vi "PH_HamamatsuCamera.ProcPeriodic.vi"(0 "i ref in":refnum<vi>, 3 "ms timeout (100)":i32=100, 5 "error in (no error)":errorcluster) -> (14 "i ref out":refnum<vi>, 17 "timed out":bool, 19 "error out":errorcluster)   [LabVIEW 2014, in "PH_HamamatsuCamera.lvlib"]
doc: "This method serves to periodically do things like reading values from the HW. Methods that should be executed periodically should be called from THIS methode. Add code here."
uses:
  PH_HamamatsuCamera.lvlib
  PH_StatusHandler/PH_StatusHandler.Status.ctl
  PH_Cam_BaseClass/PH_Cam_BaseClass.lvlib
  CSCore/BaseProcess/BaseProcess.lvlib
  PH_StatusHandler/PH_StatusHandler.lvlib
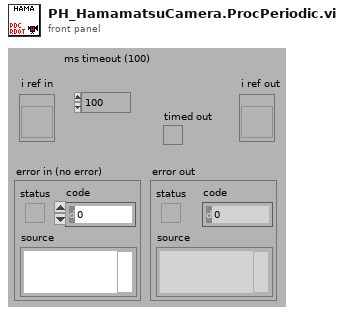
[diagram p1: front panel]
types:
  T1 = typedef "PH_Cam_BaseClass.lvlib/PH_Cam_BaseClass.i attribute.ctl" = cluster{"Gui Refs":T2, "Cam":cluster{"Source Notifier":refnum<notifier>, "Error":errorcluster, "Camera ID":string}, "Images":cluster{"Cam":T3, "Operation":T3, "PSDB":T3}, "Window Image":cluster{"Indicate Image":bool, "Window No.":i32, "Scale Facor":dbl, "Center Cross":bool, "Subtract Backgr":bool, "CoG":bool, "Color Palette":cluster{"Red":u8, "Green":u8, "Blue":u8}[], "Image On":bool}, "Default Prdc Int":i32, "Performance":cluster{"on":bool, "Timestamp Last Frame":i32}, "Histogram":cluster{"on":bool, "Mapping":bool}, "Save Image":cluster{"Save":bool, "File refnum":refnum<file>}, "Setting Service ID":i32, "Screen":cluster{"x-resolution":i16, "y-resolution":i16}, "On":bool, "Constructor finished":bool, "configured":bool}
  T2 = typedef "PH_Cam_BaseClass.lvlib/PH_Cam_BaseClass.GUI Refs.ctl" = cluster{"Frame Rate":refnum<vi>, "Get Frame Rate":refnum<vi>, "Show Image":refnum<vi>, "Get Histogram":refnum<vi>, "Mapping":refnum<vi>, "Histogram":refnum<vi>, "Center Cross":refnum<vi>, "Center of Gravity":refnum<vi>, "Scale Factor [%]":refnum<vi>, "Save Image":refnum<vi>, "Palette":refnum<vi>, "Subtract Background":refnum<vi>, "Cam Error":refnum<vi>, "On":refnum<vi>, "Cam List":refnum<vi>}
  T3 = typedef "IMAQ Image.ctl" = refnum<image>
  T4 = typedef "PH_StatusHandler.lvlib/PH_StatusHandler.Status.ctl" = i16
  T5 = typedef "PH_Cam_BaseClass.lvlib/PH_Cam_BaseClass.Settings.ctl" = cluster{"Cam ID":string, "Gain":dbl, "Brightness":dbl, "Shutter":dbl, "Mode":i32}
  T6 = typedef "PH_HamamatsuCamera.lvlib/PH_HamamatsuCamera.i attribute.ctl" = cluster{"Gui Refs":cluster{"Camera Details":refnum<vi>, "ROI":refnum<vi>, "Set ROI to Maximum":refnum<vi>, "Trigger Parameters":refnum<vi>, "Brightness":refnum<vi>, "Shutter":refnum<vi>, "Gain":refnum<vi>, "Trigger Timeout":refnum<vi>, "Trigger Polarity":refnum<vi>, "Trigger Mode":refnum<vi>, "Parameters":refnum<vi>, "Set Cam Parameter":refnum<vi>, "Parameter to set":refnum<vi>, "Value to set":refnum<vi>}, "Cam":cluster{"Handle":i32, "Details":cluster{"Model":string, "Camera ID":string, "Firmware":string}, "Buffer Info":cluster{"height":u32, "width":u32, "datatype":u32}}, "H Offset":cluster{"Value":i32, "Minimum":i32, "Maximum":i32, "Increment":i32}, "V Offset":cluster{"Value":i32, "Minimum":i32, "Maximum":i32, "Increment":i32}, "H Width":cluster{"Value":i32, "Minimum":i32, "Maximum":i32, "Increment":i32}, "V Width":cluster{"Value":i32, "Minimum":i32, "Maximum":i32, "Increment":i32}, "Trigger Parameters":T7, "Trigger Timeout":u32, "Parameters":T8[], "Indicees Cam Parameters":cluster{"Brightness":i32, "Shutter":i32, "Gain":i32}, "Wanted Values":cluster{"Trigger Settings":T7[], "ROI":T9[], "Parameter":cluster{"Name":string, "Value":dbl}[]}}
  T7 = typedef "PH_HamamatsuCamera.lvlib/PH_HamamatsuCamera.Trigger Parameter.ctl" = cluster{"Mode":u32, "Polarity":u32, "Times":u32, "Delay":dbl}
  T8 = typedef "PH_HamamatsuCamera.lvlib/PH_HamamatsuCamera.Parameter Set.ctl" = cluster{"Parameter":string, "Value":dbl, "Writable":bool, "Range":cluster{"min":dbl, "max":dbl, "step":dbl}, "Default":dbl, "Value Names":cluster{"Name":string, "Value":dbl}[], "Text Values":bool}
  T9 = typedef "PH_HamamatsuCamera.lvlib/PH_HamamatsuCamera.ROI.ctl" = cluster{"Horizontal Offset":i32, "Vertical Offset":i32, "Horizontal Width":i32, "Vertical Width":i32}
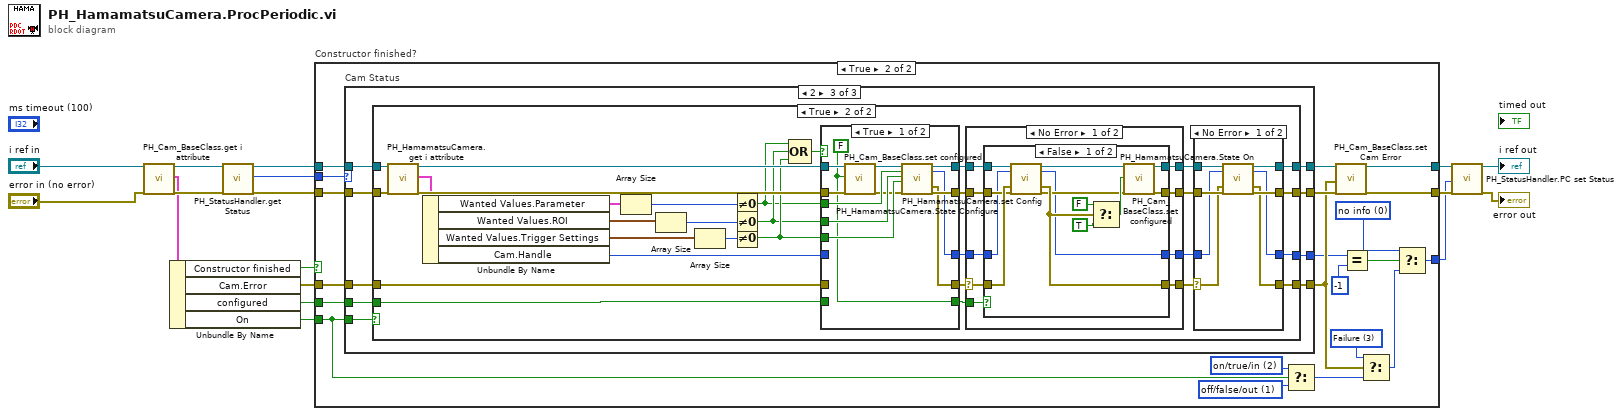
[diagram p0: block diagram]
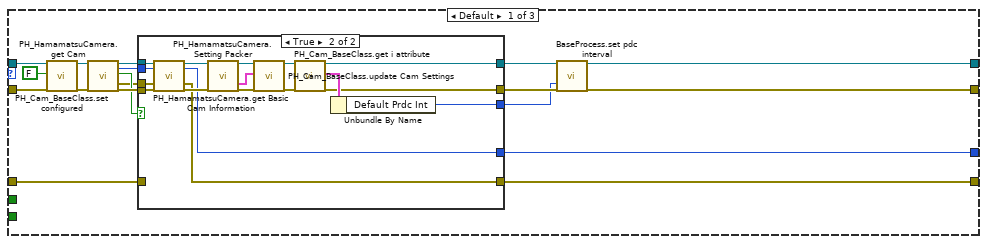
[diagram p3: hidden frame]
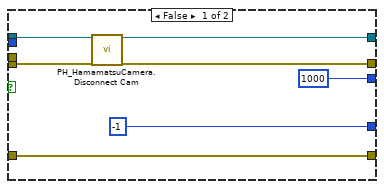
[diagram p4: hidden frame]
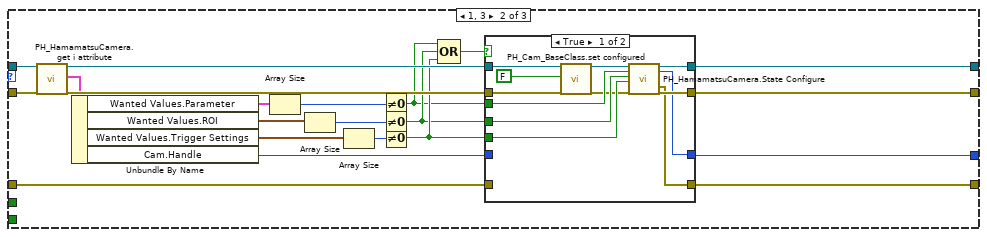
[diagram p5: hidden frame]
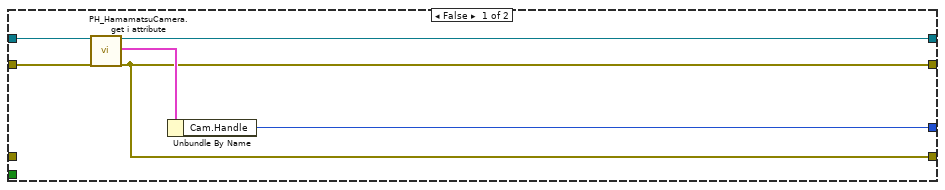
[diagram p7: hidden frame]
diagram:
  n1 = call "PH_Cam_BaseClass.get i attribute.vi"("i ref in"="i ref in", "error in (no error)"="error in (no error)") -> ("i ref out"=w3:refnum<vi>, "i attribute"=w16:T1, "error out"=w17:errorcluster)  [unwired: 15 in]
  n2 = Unbundle By Name(w16) -> ("Constructor finished"=w15:bool, "Cam.Error"=w14:errorcluster, "configured"=w5:bool, "On"=w11:bool)
  n3 = call "PH_StatusHandler.get Status.vi"("VI in"=w3, "error in"=w17) -> ("VI out"=w2:refnum<vi>, "Status"=w1:T4, "error out"=w4:errorcluster)  [unwired: 15 in]
  n4 = case "Constructor finished?" shown="True" w15 {
    tunnel: [w20 w37] -> w12
    tunnel: [w19 w36] -> w13
    tunnel: w4 -> [w19 w41]
    tunnel: w2 -> [w20 w40]
    tunnel: w1 -> [w18 w39]
    tunnel: w14 -> [_ w38]
    tunnel: w11 -> [_ w25]
    tunnel: [w18 w26] -> w10
    tunnel: w5 -> [_ w21]
    frame False {
    }
    frame True {
      w29 = T4 1 items=["no info", "off/false/out", "on/true/in", "Failure", "Alarm", "Status 1", "Status 2", "Status 3"] ("Cam State")
      w30 = T4 2 items=["no info", "off/false/out", "on/true/in", "Failure", "Alarm", "Status 1", "Status 2", "Status 3"] ("Cam State")
      w31 = T4 3 items=["no info", "off/false/out", "on/true/in", "Failure", "Alarm", "Status 1", "Status 2", "Status 3"] ("Cam State")
      w32 = T4 0 items=["no info", "off/false/out", "on/true/in", "Failure", "Alarm", "Status 1", "Status 2", "Status 3"] ("Cam State")
      n5 = case "Cam Status" shown="2" w39 {
        tunnel: [w54 w104 w129] -> w34
        tunnel: [w56 w103 w128] -> w33
        tunnel: w41 -> [w44 w102 w127]
        tunnel: w40 -> [w45 w100 w126]
        tunnel: [w51 w95 w125] -> w27
        tunnel: w38 -> [w47 w96 w123]
        tunnel: [w50 w94 w122] -> w24
        tunnel: w25 -> [_ _ w124]
        tunnel: w21 -> [_ _ w121]
        frame Default {
          n6 = call "PH_Cam_BaseClass.set configured.vi"("i ref in"=w45, "configured"=FALSE, "error in (no error)"=w44) -> ("i ref out"=w42:refnum<vi>, "error out"=w43:errorcluster)  [unwired: 15 in]
          n7 = call "PH_HamamatsuCamera.get Cam.vi"("i ref in"=w42, "error in"=w43) -> ("i ref out"=w59:refnum<vi>, "Handle out"=w49:i32, "Cam found"=w57:bool, "Cam Error out"=w48:errorcluster, "error out"=w58:errorcluster)  [unwired: 13 in]
          n8 = case shown="True" w57 {
            tunnel: w59 -> [w64 w83]
            tunnel: w58 -> [w63 w82]
            tunnel: [w62 w75] -> w53
            tunnel: [w61 w71] -> w55
            tunnel: [1000 ("Default Prdc Int") w74] -> w52
            tunnel: [w65 w70] -> w51
            tunnel: [-1 ("Cam Handle out") w67] -> w50
            tunnel: w49 -> [_ w69]
            tunnel: w48 -> [_ w68]
            tunnel: w47 -> [w65 _]
            frame False {
              n9 = call "PH_HamamatsuCamera.Disconnect Cam.vi"("VI in"=w64, "error in (no error)"=w63) -> ("VI out"=w62:refnum<vi>, "error out"=w61:errorcluster)  [unwired: 16 in]
            }
            frame True {
              n10 = call "PH_HamamatsuCamera.get Basic Cam Information.vi"("i ref in"=w83, "Cam Handle in"=w69, "Cam Error in"=w68, "error in (no error)"=w82) -> ("i ref out"=w81:refnum<vi>, "Cam Handle out"=w67:i32, "Cam Error out"=w70:errorcluster, "error out"=w79:errorcluster)  [unwired: 12 in]
              n11 = call "PH_HamamatsuCamera.Setting Packer.vi"("i ref in"=w81, "error in (no error)"=w79) -> ("i ref out"=w80:refnum<vi>, "Cam Settings"=w77:T5, "error out"=w78:errorcluster)  [unwired: 15 in]
              n12 = call "PH_Cam_BaseClass.update Cam Settings.vi"("VI in"=w80, "Cam Settings In"=w77, "error in (no error)"=w78) -> ("VI out"=w76:refnum<vi>, "error out"=w72:errorcluster)  [unwired: 15 in]
              n13 = call "PH_Cam_BaseClass.get i attribute.vi"("i ref in"=w76, "error in (no error)"=w72) -> ("i ref out"=w75:refnum<vi>, "i attribute"=w73:T1, "error out"=w71:errorcluster)  [unwired: 15 in]
              n14 = Unbundle By Name(w73) -> ("Default Prdc Int"=w74:i32)
            }
          }
          n15 = call "BaseProcess.set pdc interval.vi"("i ref in"=w53, "PeriodicInterval [ms]"=w52, "error in (no error)"=w55) -> ("i ref out"=w54:refnum<vi>, "error out"=w56:errorcluster)  [unwired: 14 in, 1 out]
        }
        frame 1, 3 {
          n16 = call "PH_HamamatsuCamera.get i attribute.vi"("i ref in"=w100, "error in (no error)"=w102) -> ("i ref out"=w99:refnum<vi>, "i attribute"=w98:T6, "error out"=w101:errorcluster)  [unwired: 15 in]
          n17 = Unbundle By Name(w98) -> ("Wanted Values.Parameter"=w97:cluster{"Name":string, "Value":dbl}[], "Wanted Values.ROI"=w93:T9[], "Wanted Values.Trigger Settings"=w92:T7[], "Cam.Handle"=w87:i32)
          n18 = Array Size(array=w97) -> (size(s)=w89:i32)
          n19 = Array Size(array=w93) -> (size(s)=w90:i32)
          n20 = Array Size(array=w92) -> (size(s)=w91:i32)
          n21 = Not Equal To 0?(x=w89) -> (x != 0?=w84:bool)
          n22 = Not Equal To 0?(x=w90) -> (x != 0?=w85:bool)
          n23 = Not Equal To 0?(x=w91) -> (x != 0?=w86:bool)
          n24 = Compound Arithmetic op=OR(w84, w85, w86) -> (w88:bool)
          n25 = case shown="True" w88 {
            tunnel: [w116 w120] -> w104
            tunnel: [w115 w119] -> w103
            tunnel: [w114 w118] -> w95
            tunnel: w101 -> [w108 w119]
            tunnel: w99 -> [w107 w120]
            tunnel: w96 -> [_ w118]
            tunnel: [w113 w117] -> w94
            tunnel: w87 -> [_ w117]
            tunnel: w86 -> [w110 _]
            tunnel: w85 -> [w111 _]
            tunnel: w84 -> [w112 _]
            frame True {
              n26 = call "PH_Cam_BaseClass.set configured.vi"("i ref in"=w107, "configured"=FALSE, "error in (no error)"=w108) -> ("i ref out"=w106:refnum<vi>, "error out"=w105:errorcluster)  [unwired: 15 in]
              n27 = call "PH_HamamatsuCamera.State Configure.vi"("VI in"=w106, "Parameter changed"=w112, "ROI changed"=w111, "Trigger Sets changed"=w110, "error in (no error)"=w105) -> ("VI out"=w116:refnum<vi>, "Cam Handle out"=w113:i32, "Cam Error"=w114:errorcluster, "error out"=w115:errorcluster)  [unwired: 11 in]
            }
            frame False {
            }
          }
        }
        frame 2 {
          n28 = case shown="True" w124 {
            tunnel: [w133 w166] -> w129
            tunnel: [w132 w165] -> w128
            tunnel: w127 -> [w130 w148]
            tunnel: w126 -> [w131 w149]
            tunnel: [w132 w164] -> w125
            tunnel: [w134 w146] -> w122
            tunnel: w123 -> [_ w147]
            tunnel: w121 -> [_ w139]
            frame False {
              n29 = call "PH_HamamatsuCamera.get i attribute.vi"("i ref in"=w131, "error in (no error)"=w130) -> ("i ref out"=w133:refnum<vi>, "i attribute"=w135:T6, "error out"=w132:errorcluster)  [unwired: 15 in]
              n30 = Unbundle By Name(w135) -> ("Cam.Handle"=w134:i32)
            }
            frame True {
              n31 = call "PH_HamamatsuCamera.get i attribute.vi"("i ref in"=w149, "error in (no error)"=w148) -> ("i ref out"=w162:refnum<vi>, "i attribute"=w161:T6, "error out"=w163:errorcluster)  [unwired: 15 in]
              n32 = Unbundle By Name(w161) -> ("Wanted Values.Parameter"=w160:cluster{"Name":string, "Value":dbl}[], "Wanted Values.ROI"=w159:T9[], "Wanted Values.Trigger Settings"=w158:T7[], "Cam.Handle"=w153:i32)
              n33 = Array Size(array=w160) -> (size(s)=w155:i32)
              n34 = Array Size(array=w159) -> (size(s)=w156:i32)
              n35 = Array Size(array=w158) -> (size(s)=w157:i32)
              n36 = Not Equal To 0?(x=w155) -> (x != 0?=w150:bool)
              n37 = Not Equal To 0?(x=w156) -> (x != 0?=w151:bool)
              n38 = Not Equal To 0?(x=w157) -> (x != 0?=w152:bool)
              n39 = Compound Arithmetic op=OR(w150, w151, w152) -> (w154:bool)
              n40 = case shown="True" w154 {
                tunnel: [w208 w213] -> w145
                tunnel: [w207 w212] -> w144
                tunnel: [w206 w211] -> w141
                tunnel: w163 -> [w201 w212]
                tunnel: w162 -> [w200 w213]
                tunnel: w147 -> [_ w211]
                tunnel: [w205 w210] -> w140
                tunnel: w153 -> [_ w210]
                tunnel: w152 -> [w202 _]
                tunnel: w151 -> [w203 _]
                tunnel: w150 -> [w204 _]
                tunnel: [w197 w209] -> w138
                tunnel: w139 -> [_ w209]
                frame True {
                  w197 = FALSE ("configured")
                  n41 = call "PH_Cam_BaseClass.set configured.vi"("i ref in"=w200, "configured"=w197, "error in (no error)"=w201) -> ("i ref out"=w199:refnum<vi>, "error out"=w198:errorcluster)  [unwired: 15 in]
                  n42 = call "PH_HamamatsuCamera.State Configure.vi"("VI in"=w199, "Parameter changed"=w204, "ROI changed"=w203, "Trigger Sets changed"=w202, "error in (no error)"=w198) -> ("VI out"=w208:refnum<vi>, "Cam Handle out"=w205:i32, "Cam Error"=w206:errorcluster, "error out"=w207:errorcluster)  [unwired: 11 in]
                }
                frame False {
                }
              }
              n43 = case shown="No Error" w141 {
                selector: w141 -> [w170 w194]
                tunnel: [w175 w193] -> w136
                tunnel: [w169 w194] -> w137
                tunnel: [w174 w195] -> w142
                tunnel: w144 -> [w173 w195]
                tunnel: [w172 w196] -> w143
                tunnel: w145 -> [w171 w196]
                tunnel: w138 -> [w168 _]
                tunnel: w140 -> [w167 w193]
                frame No Error {
                  n44 = case shown="False" w168 {
                    tunnel: [w176 w189] -> w175
                    tunnel: [w185 w191] -> w174
                    tunnel: w173 -> [w181 w191]
                    tunnel: [w184 w192] -> w172
                    tunnel: w171 -> [w179 w192]
                    tunnel: w170 -> [w182 w190]
                    tunnel: [w183 w190] -> w169
                    tunnel: w167 -> [w178 w189]
                    frame False {
                      n45 = call "PH_HamamatsuCamera.set Config.vi"("VI in"=w179, "Cam Handle in"=w178, "Cam Error in"=w182, "error in"=w181) -> ("VI out"=w177:refnum<vi>, "Cam Handle out"=w176:i32, "Cam Error out"=w183:errorcluster, "error out"=w180:errorcluster)  [unwired: 12 in]
                      n46 = Select(t=FALSE, s=w183, f=TRUE ("configured")) -> (s? t:f=w186:bool)
                      n47 = call "PH_Cam_BaseClass.set configured.vi"("i ref in"=w177, "configured"=w186, "error in (no error)"=w180) -> ("i ref out"=w184:refnum<vi>, "error out"=w185:errorcluster)  [unwired: 15 in]
                    }
                    frame True {
                    }
                  }
                }
                frame Error {
                }
              }
              n48 = case shown="No Error" w137 {
                selector: w137 -> [w215 w223]
                tunnel: [w221 w225] -> w166
                tunnel: [w220 w224] -> w165
                tunnel: [w219 w223] -> w164
                tunnel: w142 -> [w218 w224]
                tunnel: w143 -> [w217 w225]
                tunnel: w136 -> [w216 w222]
                tunnel: [w214 w222] -> w146
                frame No Error {
                  n49 = call "PH_HamamatsuCamera.State On.vi"("VI in"=w217, "Cam Handle in"=w216, "Cam Error in"=w215, "error in (no error)"=w218) -> ("VI out"=w221:refnum<vi>, "Cam Handle"=w214:i32, "Cam Error"=w219:errorcluster, "error out"=w220:errorcluster)  [unwired: 12 in]
                }
                frame Error {
                }
              }
            }
          }
        }
      }
      n50 = Select(t=w30, s=w25, f=w29) -> (s? t:f=w28:T4)
      n51 = call "PH_Cam_BaseClass.set Cam Error.vi"("VI in"=w34, "Cam Error"=w27, "error in"=w33) -> ("VI out"=w37:refnum<vi>, "error out"=w36:errorcluster)  [unwired: 15 in]
      n52 = Equal?(x=w24, y=-1) -> (x = y?=w22:bool)
      n53 = Select(t=w31, s=w27, f=w28) -> (s? t:f=w35:T4)
      n54 = Select(t=w32, s=w22, f=w35) -> (s? t:f=w26:T4)
    }
  }
  n55 = call "PH_StatusHandler.PC set Status.vi"("i ref in"=w12, "Status"=w10, "error in (no error)"=w13) -> ("i ref out"=→"i ref out":refnum<vi>, "error out"=→"error out":errorcluster)  [unwired: 15 in]
